vi "EMG - Wavelet.vi"() -> ()   [LabVIEW 2013]
panel:
  out "Lokacija sacuvanog fajla na racunaru":path
  out "Entropija":dbl[](array[numeric]) caption="entropy" format="%.2f"
  out "Koeficijenti cvorova":cluster{"koeficijent":dbl[]}[](array[cluster]) caption="node coeffs"
  out "Signal nakon wavelet analize":waveform(dbl)(graph)
  out "Signal pre analize":waveform(dbl)[](graph)
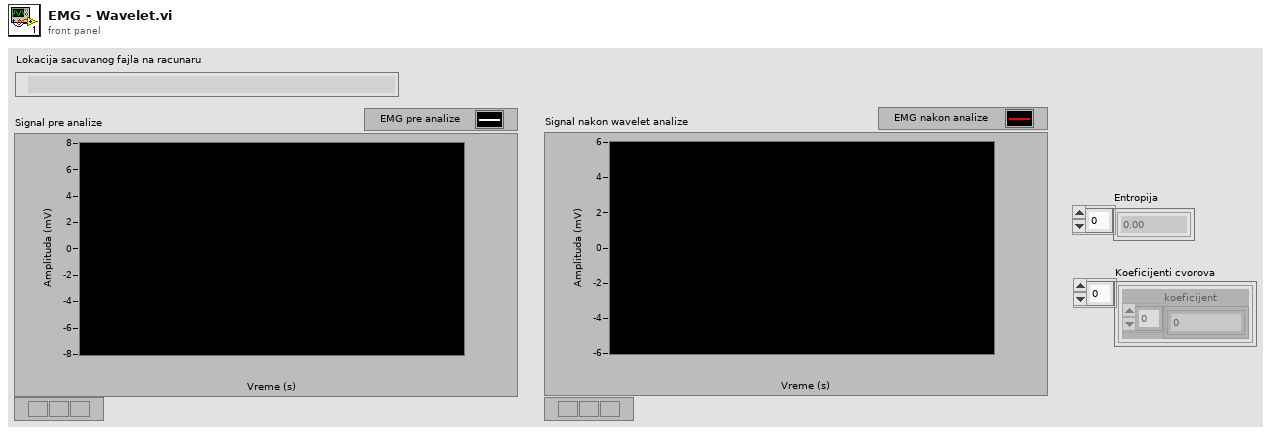
[diagram p1: front panel]
types:
  T1 = enum16{"open", "open or create", "create or replace", "create", "open (read-only)"}
  T2 = enum16{"open", "replace", "create", "open or create", "replace or create", "replace or create with confirmation"}
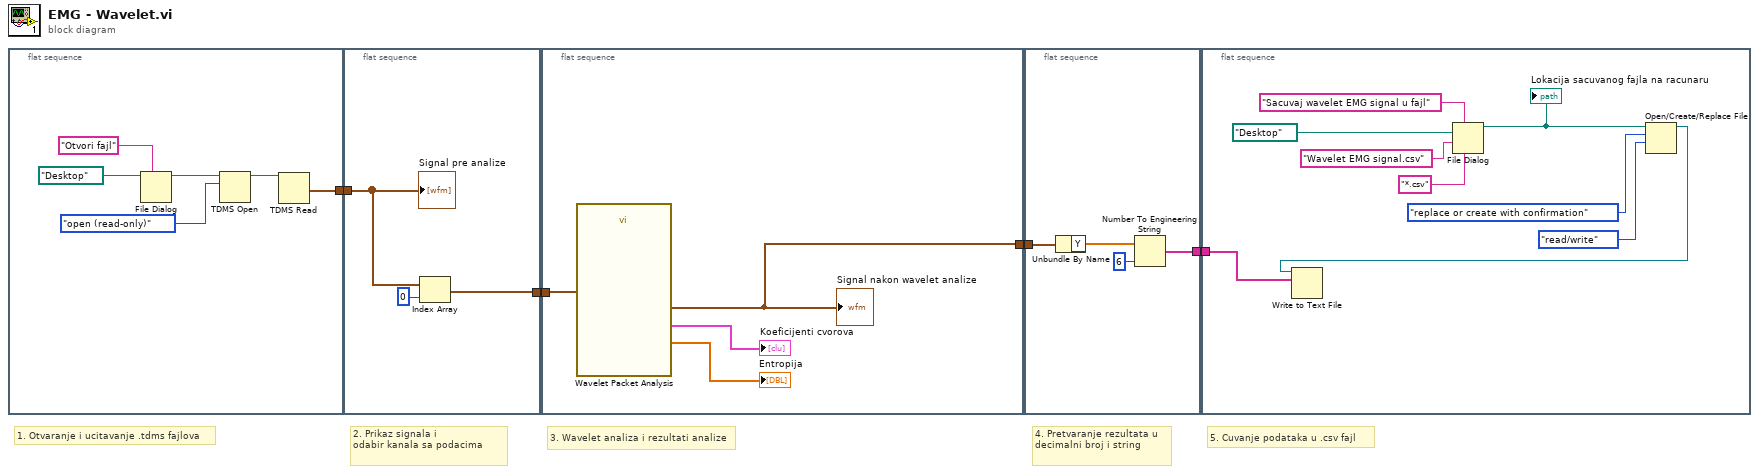
[diagram p0: block diagram]
diagram:
  # "5. Cuvanje podataka u .csv fajl"
  # "4. Pretvaranje rezultata u decimalni broj i string"
  # "3. Wavelet analiza i rezultati analize"
  # "2. Prikaz signala i \nodabir kanala sa podacima"
  # "1. Otvaranje i ucitavanje .tdms fajlova"
  n1 = flat-sequence {
    tunnel: [w6] -> w4
    frame #0 {
      n2 = File Dialog(7:"Otvori fajl" ("prompt"), 11:path "/Desktop" ("start path")) -> (3:w8:path)  [unwired: 2 in, 6 out]
      n3 = TDMS Open(10:T1."open (read-only)" ("operation (0:open)"), 11:w8) -> (3:w9:refnum<k34>)  [unwired: 5 in, 1 out]
      n4 = TDMS Read(0:w9) -> (10:w6:waveform(dbl)[])  [unwired: 7 in, 5 out]
    }
  }
  n5 = flat-sequence {
    tunnel: w4 -> [w13]
    tunnel: [w11] -> w1
    frame #0 {
      n6 = Index Array(array=w13, index=0) -> (element=w11:waveform(dbl))
      "Signal pre analize" <- w13
    }
  }
  n7 = flat-sequence {
    tunnel: [w17] -> w2
    tunnel: w1 -> [w14]
    frame #0 {
      n8 = call "Wavelet Packet Analysis"("Signal"=w14) -> ("entropy"=→"Entropija":dbl[], "node coeffs"=→"Koeficijenti cvorova":cluster{"node coef":dbl[]}[], "Reconstruction"=w17:waveform(dbl))  [unwired: 6 in, 2 out]
      "Signal nakon wavelet analize" <- w17
    }
  }
  n9 = flat-sequence {
    tunnel: [w21] -> w3
    tunnel: w2 -> [w20]
    frame #0 {
      n10 = Unbundle By Name ("Get Waveform Components")(w20) -> ("Y"=w19:dbl[])
      n11 = Number To Engineering String(2:i16 6 ("precision (6)"), 4:w19) -> (0:w21:string[])  [unwired: 2 in]
    }
  }
  n12 = flat-sequence {
    tunnel: w3 -> [w23]
    frame #0 {
      n13 = File Dialog(6:"*.csv" ("pattern (all files)"), 7:"Sacuvaj wavelet EMG signal u fajl" ("prompt"), 9:"Wavelet EMG signal.csv" ("default name"), 11:path "/Desktop" ("start path")) -> (3:w25:path)  [unwired: 1 in, 5 out]
      "Lokacija sacuvanog fajla na racunaru" <- w25
      n14 = Open/Create/Replace File(file path (use dialog)=w25, operation (0:open)=T2."replace or create with confirmation", access (0:read/write)=enum16{"read/write", "read-only", "write-only"}."read/write") -> (refnum out=w22:refnum<file>)  [unwired: 3 in, 2 out]
      n15 = Write to Text File(file (use dialog)=w22, text=w23) -> ()  [unwired: 2 in, 3 out]
    }
  }
